vi "2283_controlDeElevador.vi"(0 "Cluster Niveles":T1) -> (2 "Output elevador":dbl)   [LabVIEW 2014]
uses:
  <vilib>/Rock Robotics/WPI/Solenoid/WPI_SolenoidValue.ctl
  Secuencia de Recoger Control.ctl
  DevRefs Global.vi
  Grip Overwrite Global.vi
  Cuernitos Global.vi
panel:
  in  "Margen de Error Secuencia de Recoger":dbl=50.0 format="%#_13g"
  in  "Nivel Cargar":dbl=60.0 format="%#_13g"
  in  "Nivel 1 Caja":dbl=225.0 format="%#_13g"
  in  "Nivel 2 Cajas":dbl=385.0 format="%#_13g"
  in  "Nivel 3 Cajas":dbl=607.0 format="%#_13g"
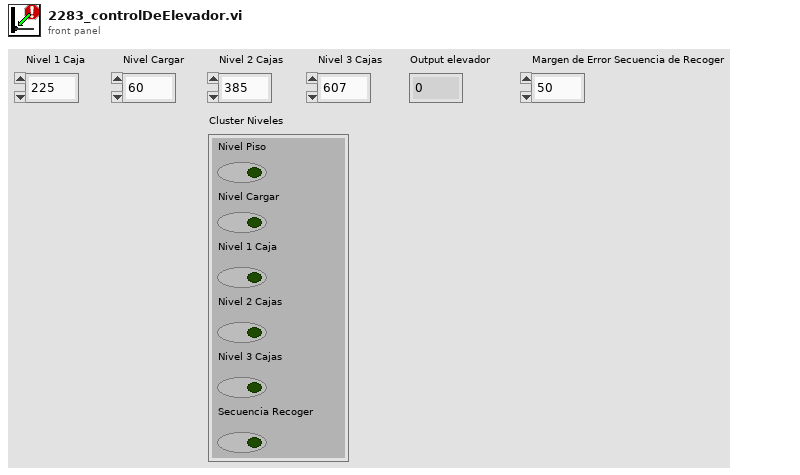
[diagram p1: front panel]
types:
  T1 = cluster{"Nivel Piso":bool, "Nivel Cargar":bool, "Nivel 1 Caja":bool, "Nivel 2 Cajas":bool, "Nivel 3 Cajas":bool, "Secuencia Recoger":bool}
  T2 = typedef "WPI_SolenoidDevRef.ctl" = cluster{"DevStatus":errorcluster, "Pneumatics Control Module":u8, "Forward Solenoid Channel":T3, "Reverse Solenoid Channel":T3}
  T3 = typedef "WPI_SolenoidChannel.ctl" = enum8{"Solenoid 0", "Solenoid 1", "Solenoid 2", "Solenoid 3", "Solenoid 4", "Solenoid 5", "Solenoid 6", "Solenoid 7", "Invalid"}
  T4 = typedef "WPI_MotorControlDeviceRef.ctl" = cluster{"DeviceStatus":errorcluster, "Type":T5, "PWM":cluster{"Controller":T6, "PWM Channel":T7, "DeadBand":T8}, "CAN":cluster{"Device Number":u8, "Control Mode":T9, "Semaphore":T10, "Max Vout":dbl, "TalonSRX Control Mode":T11}, "Invert":bool, "TransformRef":T12, "InvTransformRef":T12}
  T5 = typedef "WPI_MotorControlType.ctl" = enum16{"PWM", "CAN", "CANTalonSRX"}
  T6 = typedef "FPGA_TypedefDigitalModule.ctl" = enum16{"Controller 1"}
  T7 = typedef "FPGA_DIOPWMChannel.ctl" = enum8{"PWM 0", "PWM 1", "PWM 2", "PWM 3", "PWM 4", "PWM 5", "PWM 6", "PWM 7", "PWM 8", "PWM 9", "PWM MXP 0", "PWM MXP 1", "PWM MXP 2", "PWM MXP 3", "PWM MXP 4", "PWM MXP 5", "PWM MXP 6", "PWM MXP 7", "PWM MXP 8", "PWM MXP 9", "Invalid"}
  T8 = typedef "WPI_PWMDeadband.ctl" = cluster{"Name":string, "maxPositivePwm":i32, "minPositivePwm":i32, "centerPwm":i32, "maxNegativePwm":i32, "minNegativePwm":i32, "angularRange":u16}
  T9 = typedef "WPI_CANJaguar_ControlMode.ctl" = enum8{"Percent VBus", "Current", "Speed", "Position", "Voltage"}
  T10 = typedef "Semaphore RefNum" = refnum<k1>
  T11 = typedef "WPI_CANTalonSRX_APIControlMode.ctl" = enum8{"Percent VBus", "Speed", "Position", "Slave", "Unchanged / Invalid"}
  T12 = typedef "WPI_PWMTransform_ConPane.ctl" = refnum<vi>
  T13 = typedef "WPI_CompressorDevRef.ctl" = cluster{"DevStatus":errorcluster, "Pneumatics Control Module":u8}
  T14 = typedef "WPI_SwitchDevRef.ctl" = cluster{"DevStatus":errorcluster, "DIO Channel":T15, "Controller":T6, "CntIndex":T16, "Normally Closed":bool}
  T15 = typedef "FPGA_DIOChannel.ctl" = enum8{"DIO 0", "DIO 1", "DIO 2", "DIO 3", "DIO 4", "DIO 5", "DIO 6", "DIO 7", "DIO 8", "DIO 9", "DIO MXP 0", "DIO MXP 1", "DIO MXP 2", "DIO MXP 3", "DIO MXP 4", "DIO MXP 5", "DIO MXP 6", "DIO MXP 7", "DIO MXP 8", "DIO MXP 9", "DIO MXP 10", "DIO MXP 11", "DIO MXP 12", "DIO MXP 13", "DIO MXP 14", "DIO MXP 15", "Invalid"}
  T16 = typedef "FPGA_CounterCtrSystemIndex.ctl" = enum8{"Ctr 0", "Ctr 1", "Ctr 2", "Ctr 3", "Ctr 4", "Ctr 5", "Ctr 6", "Ctr 7", "Invalid"}
  T17 = typedef "WPI_GyroDevRef.ctl" = cluster{"DevStatus":errorcluster, "Analog Module":T18, "Analog Channel":T19, "Offset":dbl, "Gain (VoltsPerDegree/Second)":dbl}
  T18 = typedef "FPGA_TypedefAnalogModule.ctl" = enum16{"Controller 1"}
  T19 = typedef "FPGA_AIChannel.ctl" = enum8{"AI 0", "AI 1", "AI 2", "AI 3", "AI MXP 0", "AI MXP 1", "AI MXP 2", "AI MXP 3", "Invalid"}
  T20 = typedef "WPI_JoystickDevRef.ctl" = cluster{"Device":T21}
  T21 = typedef "WPI_JoystickDeviceEnum.ctl" = enum16{"USB 0", "USB 1", "USB 2", "USB 3", "USB 4", "USB 5"}
  T22 = typedef "WPI_AccelerometerDevRef.ctl" = cluster{"DevStatus":errorcluster, "Controller":T18, "Scaling":T23, "Analog Channels":T24, "I2C Bus":T25, "SPI Bus":T26, "Accel Range":T27, "ADXL345 Axes":T28, "Handle":i32, "Device Address":u8, "Accel Type":enum16{"Analog", "ADXL345 I2C", "ADXL345 SPI", "Internal"}}
  T23 = typedef "WPI_AccelerometerScaling.ctl" = cluster{"Gain (VoltsPerG)":dbl, "Center Voltage":dbl}
  T24 = typedef "WPI_AccelerometerAnalogChannels.ctl" = cluster{"X-Axis":T19, "Y-Axis":T19, "Z-Axis":T19}
  T25 = typedef "i2c_bus.ctl" = enum16{"I2C On-Board", "I2C MXP", "Invalid"}
  T26 = typedef "spi_bus.ctl" = enum16{"SPI On-Board, CS0", "SPI On-Board, CS1", "SPI On-Board, CS2", "SPI On-Board, CS3", "SPI MXP", "Invalid"}
  T27 = typedef "ADXL345 Range.ctl" = u8
  T28 = typedef "WPI_AccelerometerADXL345 Axes.ctl" = cluster{"X-Axis":bool, "Y-Axis":bool, "Z-Axis":bool}
  T29 = typedef "WPI_ServoDeviceRef.ctl" = cluster{"DeviceStatus":errorcluster, "Controller":T6, "PWM Channel":T7, "DeadBand":T8}
  T30 = typedef "WPI_EncoderDevRef.ctl" = cluster{"DevStatus":errorcluster, "EncoderIndex":T31, "CounterIndex":T16, "DistancePerCount":dbl, "Decoding Type":T32}
  T31 = typedef "FPGA_EncoderIdx.ctl" = enum8{"Enc 0", "Enc 1", "Enc 2", "Enc 3", "Enc 4", "Enc 5", "Enc 6", "Enc 7", "Invalid"}
  T32 = typedef "WPI_EncoderType.ctl" = enum16{"1x", "2x", "4x"}
  T33 = typedef "WPI_I2CDevRef.ctl" = cluster{"DevStatus":errorcluster, "Controller":T6, "Device Address":u8, "Handle":i32, "I2C Bus":T25}
  T34 = cluster{"Solenoide Cuernito Izquierdo":T2, "Solenoide Cuernito Derecho":T2, "Gripper":T2, "CAN Derecho Adelante":T4, "CAN Derecho Atras":T4, "CAN Izquierdo Atras":T4, "CAN Izquierdo Adelante":T4, "Compresora":T13, "Elevador Abajo":T14, "Elevador Abajo 2":T14, "Elevador Arriba":T14, "Gyro 1":T17, "Gyro 2":T17, "Joystick":T20, "Driver Station":T20, "Motor Cuernito Derecho":T4, "Motor Cuernito Izquierdo":T4, "Acelerometro":T22, "Servo":T29, "Encoder Elevador":T30, "Motor 1 Elevador":T4, "Motor 2 Elevador":T4, "Arduino I2C":T33, "LIDAR I2C":T33}
  T35 = typedef "WPI_SolenoidValue.ctl" = enum16{"Off", "On", "Forward", "Reverse"}
  T36 = typedef "Seleccion de Nivel Control.ctl" = enum16{"NA", "Nivel Piso", "Nivel Cargar", "Nivel 1 Caja", "Nivel 2 Cajas", "Nivel 3 Cajas", "Secuencia Recoger"}
  T37 = cluster{"Nivel Cargar":dbl, "Nivel 1 Caja":dbl, "Nivel 2 Cajas":dbl, "Nivel 3 Cajas":dbl}
  T38 = typedef "Secuencia de Recoger Control.ctl" = enum16{"Bajar a Suelo", "Abrir Cuernitos", "Subir a Cargar", "Stand-by"}
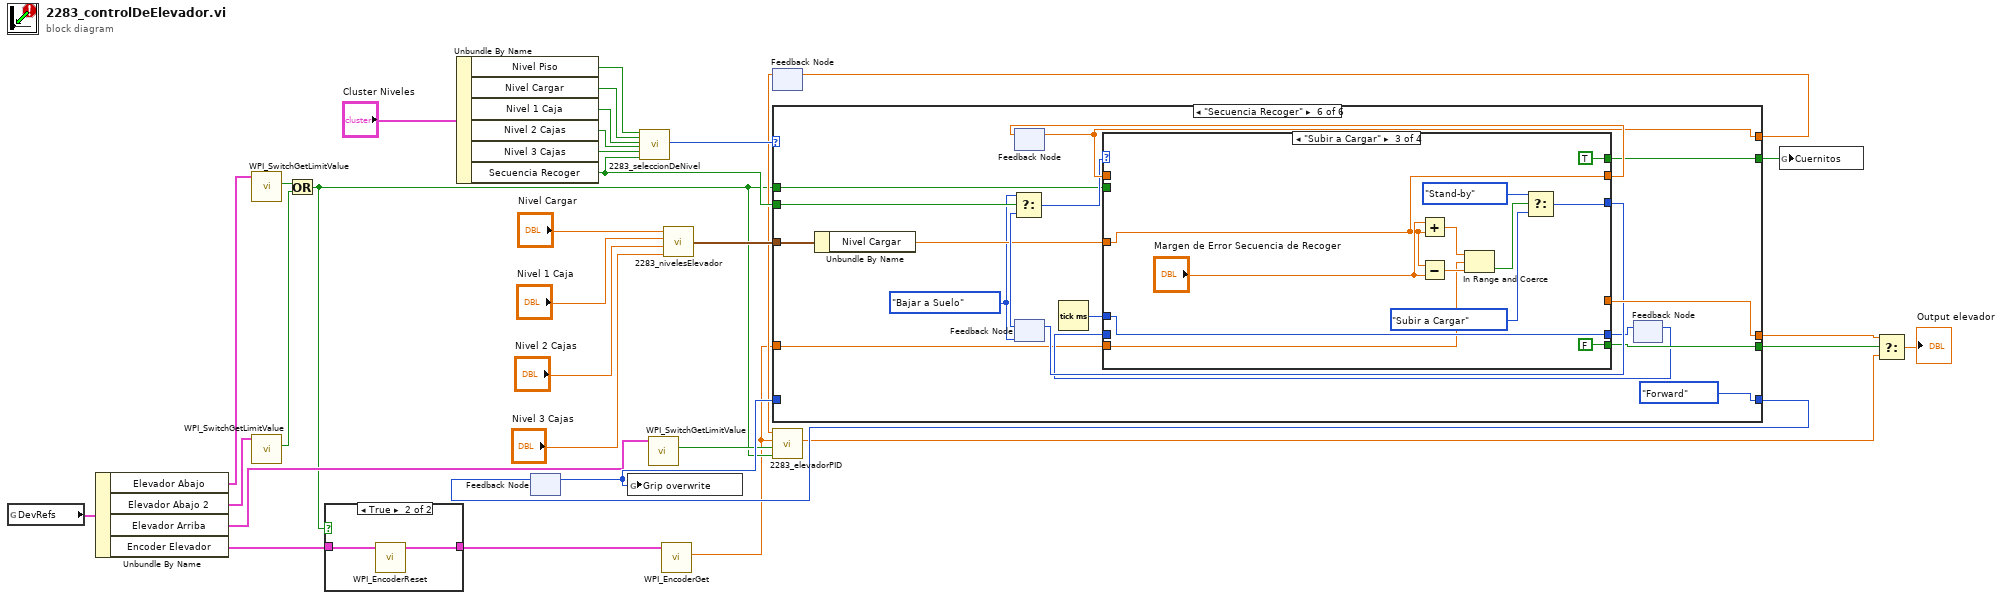
[diagram p0: block diagram]
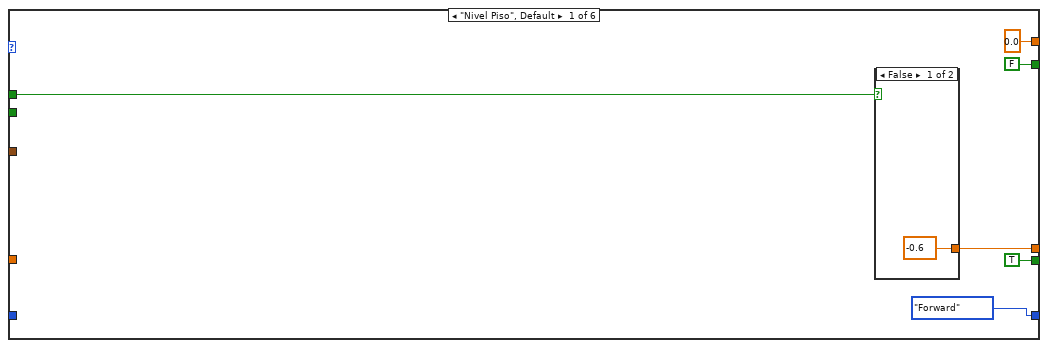
[diagram p2: hidden frame]
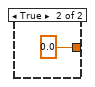
[diagram p3: hidden frame]
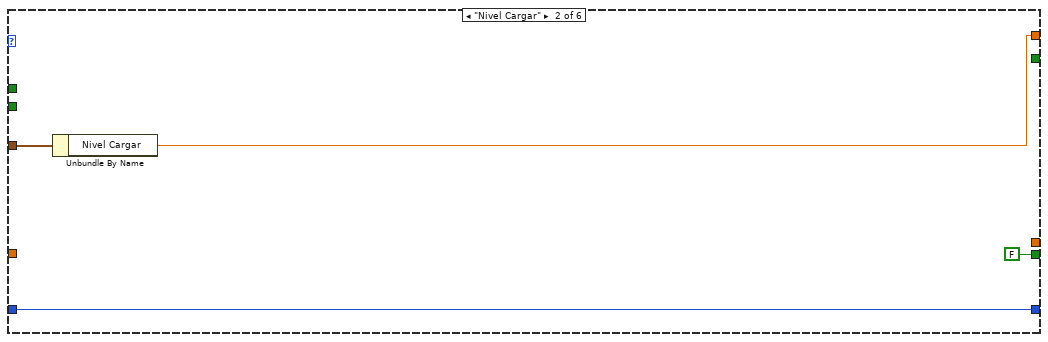
[diagram p4: hidden frame]
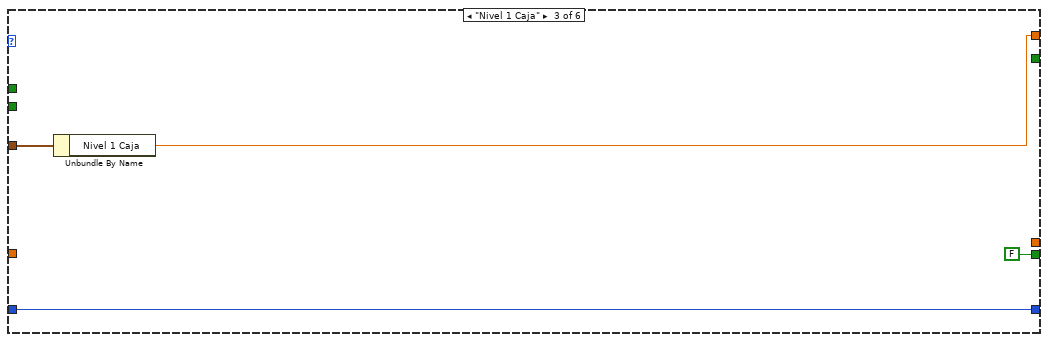
[diagram p5: hidden frame]
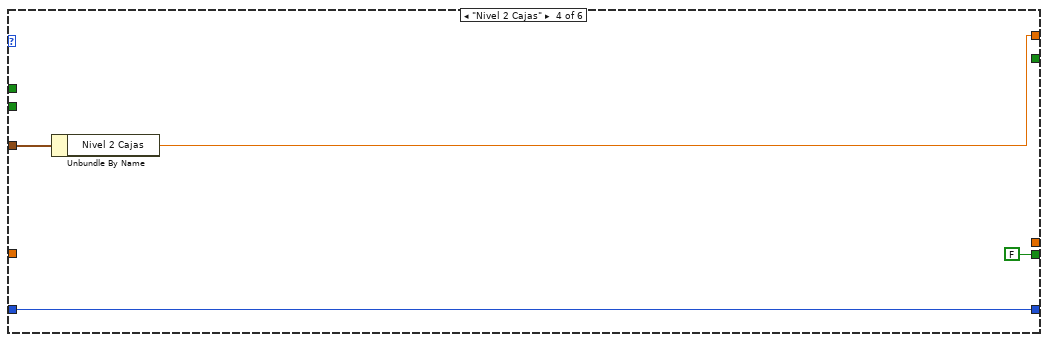
[diagram p6: hidden frame]
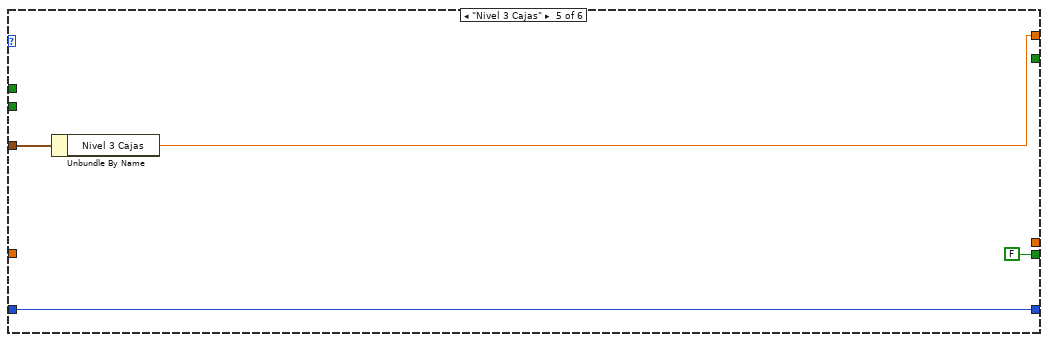
[diagram p7: hidden frame]
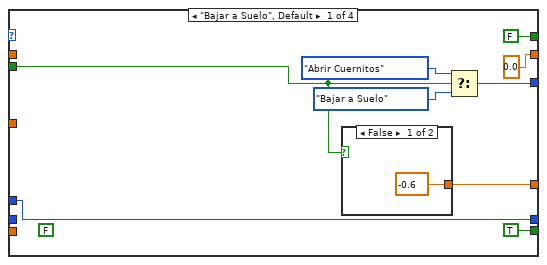
[diagram p8: hidden frame]
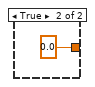
[diagram p9: hidden frame]
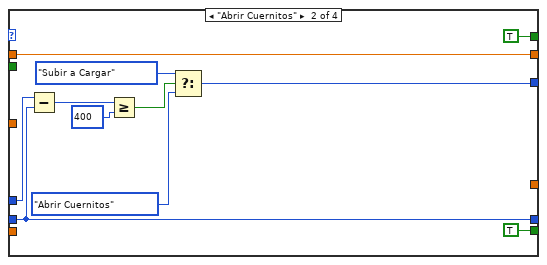
[diagram p10: hidden frame]
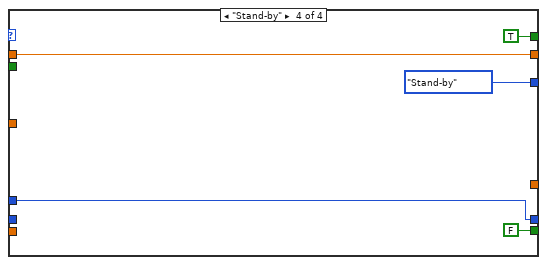
[diagram p11: hidden frame]
diagram:
  n1 = global read "DevRefs Global.vi" "DevRefs"() -> (w11:T34)
  n2 = Unbundle By Name(w11) -> ("Elevador Abajo"=w10:T14, "Elevador Abajo 2"=w9:T14, "Elevador Arriba"=w7:T14, "Encoder Elevador"=w6:T30)
  n3 = call <vilib>:"WPI_SwitchGetLimitValue.vi"("SwitchDevRef"=w10) -> ("Switch Pressed"=w22:bool)  [unwired: 8 in, 2 out]
  n4 = call <vilib>:"WPI_SwitchGetLimitValue.vi"("SwitchDevRef"=w9) -> ("Switch Pressed"=w8:bool)  [unwired: 8 in, 2 out]
  n5 = Or(x=w22, y=w8) -> (x .or. y?=w2:bool)
  n6 = case shown="True" w2 {
    tunnel: w6 -> [w34 w36]
    tunnel: [w34 w35] -> w33
    frame False {
    }
    frame True {
      n7 = call <vilib>:"WPI_EncoderReset.vi"("EncoderDevRef"=w36) -> ("EncoderDevRef"=w35:T30)  [unwired: 9 in, 1 out]
    }
  }
  n8 = Unbundle By Name("Cluster Niveles") -> ("Nivel Piso"=w17:bool, "Nivel Cargar"=w16:bool, "Nivel 1 Caja"=w15:bool, "Nivel 2 Cajas"=w14:bool, "Nivel 3 Cajas"=w13:bool, "Secuencia Recoger"=w12:bool)
  n9 = feedback #1() -> (w23:T35)  [unwired: 1 in]
  n10 = global write "Grip Overwrite Global.vi" "Grip overwrite"(w23) -> ()
  n11 = call "2283_seleccionDeNivel.vi"("Nivel Piso"=w17, "Nivel Cargar"=w16, "Nivel 1 Caja"=w15, "Nivel 2 Cajas"=w14, "Nivel 3 Cajas"=w13, "Secuencia Recoger"=w12) -> ("Nivel Deseado"=w18:T36)  [unwired: 13 in]
  n12 = call <vilib>:"WPI_SwitchGetLimitValue.vi"("SwitchDevRef"=w7) -> ("Switch Pressed"=w3:bool)  [unwired: 8 in, 2 out]
  n13 = call <vilib>:"WPI_EncoderGet.vi"("EncoderDevRef"=w33) -> ("Distance"=w1:dbl)  [unwired: 5 in, 5 out]
  n14 = call "2283_nivelesElevador.vi"("Nivel 3 cajas"="Nivel 3 Cajas", "Nivel 2 cajas"="Nivel 2 Cajas", "Nivel 1 caja"="Nivel 1 Caja", "Nivel cargar"="Nivel Cargar") -> ("output cluster"=w19:T37)
  n15 = feedback #2() -> (w4:dbl)  [unwired: 1 in]
  n16 = case shown="\"Secuencia Recoger\"" w18 {
    tunnel: [0.0 ("Nivel 1 caja") w47 w50 w54 w57 w75] -> w27
    tunnel: [w41 _ _ _ _ w78] -> w26
    tunnel: [FALSE _ _ _ _ w67] -> w21
    tunnel: [TRUE FALSE FALSE FALSE FALSE w72] -> w20
    tunnel: w12 -> [_ _ _ _ _ w68]
    tunnel: [WPI_SolenoidValue."Forward" ("Value") w48 w52 w56 w60 WPI_SolenoidValue."Forward" ("Value")] -> w24
    tunnel: w23 -> [_ w48 w52 w56 w60 _]
    tunnel: w19 -> [_ w46 w49 w55 w58 w65]
    tunnel: w2 -> [w37 _ _ _ _ w62]
    tunnel: w1 -> [_ _ _ _ _ w61]
    frame "Nivel Piso", Default {
      n17 = case shown="False" w37 {
        tunnel: [-0.6 ("upper limit") 0.0 ("upper limit")] -> w41
        frame False {
        }
        frame True {
        }
      }
    }
    frame "Nivel Cargar" {
      n18 = Unbundle By Name(w46) -> ("Nivel Cargar"=w47:dbl)
    }
    frame "Nivel 1 Caja" {
      n19 = Unbundle By Name(w49) -> ("Nivel 1 Caja"=w50:dbl)
    }
    frame "Nivel 2 Cajas" {
      n20 = Unbundle By Name(w55) -> ("Nivel 2 Cajas"=w54:dbl)
    }
    frame "Nivel 3 Cajas" {
      n21 = Unbundle By Name(w58) -> ("Nivel 3 Cajas"=w57:dbl)
    }
    frame "Secuencia Recoger" {
      w63 = Secuencia_de_Recoger_Control."Bajar a Suelo"
      n22 = Unbundle By Name(w65) -> ("Nivel Cargar"=w64:dbl)
      n23 = feedback #3() -> (w75:dbl)  [unwired: 1 in]
      n24 = feedback #4(w63) -> (w74:T38)
      n25 = Select(t=w63, s=w68, f=w74) -> (s? t:f=w73:T38)
      n26 = Tick Count (ms)() -> (millisecond timer value=w69:u32)
      n27 = feedback #5() -> (w70:u32)  [unwired: 1 in]
      n28 = case shown="\"Subir a Cargar\"" w73 {
        tunnel: w64 -> [_ _ w104 _]
        tunnel: [0.0 ("Nivel 1 caja") w100 w104 w113] -> w76
        tunnel: [w87 _ _ _] -> w78
        tunnel: [w86 w99 w108 Secuencia_de_Recoger_Control."Stand-by"] -> w77
        tunnel: w75 -> [_ w100 _ w113]
        tunnel: [FALSE ("Cuernitos") TRUE ("Cuernitos") TRUE ("Cuernitos") TRUE ("Cuernitos")] -> w67
        tunnel: [TRUE TRUE FALSE FALSE] -> w72
        tunnel: [w82 w93 w105 w116] -> w71
        tunnel: w70 -> [_ w93 _ _]
        tunnel: w69 -> [w82 w95 w105 w116]
        tunnel: w62 -> [w79 _ _ _]
        tunnel: w61 -> [_ _ w101 _]
        frame "Bajar a Suelo", Default {
          (unwired) FALSE
          n29 = case shown="False" w79 {
            tunnel: [-0.6 ("upper limit") 0.0 ("upper limit")] -> w87
            frame False {
            }
            frame True {
            }
          }
          n30 = Select(t=Secuencia_de_Recoger_Control."Abrir Cuernitos", s=w79, f=Secuencia_de_Recoger_Control."Bajar a Suelo") -> (s? t:f=w86:T38)
        }
        frame "Abrir Cuernitos" {
          n31 = Subtract(x=w95, y=w93) -> (x-y=w97:u32)
          n32 = Greater Or Equal?(x=w97, y=u32 400) -> (x >= y?=w94:bool)
          n33 = Select(t=Secuencia_de_Recoger_Control."Subir a Cargar", s=w94, f=Secuencia_de_Recoger_Control."Abrir Cuernitos") -> (s? t:f=w99:T38)
        }
        frame "Subir a Cargar" {
          n34 = Add(x="Margen de Error Secuencia de Recoger", y=w104) -> (x+y=w110:dbl)
          n35 = Subtract(x=w104, y="Margen de Error Secuencia de Recoger") -> (x-y=w112:dbl)
          n36 = In Range and Coerce(upper limit=w110, x=w101, lower limit=w112) -> (In Range?=w109:bool)  [unwired: 1 out]
          n37 = Select(t=Secuencia_de_Recoger_Control."Stand-by", s=w109, f=Secuencia_de_Recoger_Control."Subir a Cargar") -> (s? t:f=w108:T38)
        }
        frame "Stand-by" {
        }
      }
      n38 = feedback-in #3(w76) -> ()
      n39 = feedback-in #4(w77) -> ()
      n40 = feedback-in #5(w71) -> ()
    }
  }
  n41 = feedback-in #1(w24) -> ()
  n42 = feedback-in #2(w27) -> ()
  n43 = call "2283_elevadorPID.vi"("Tocando Switch abajo"=w2, "Tocando Switch Arriba"=w3, "process variable"=w1, "setpoint"=w4) -> ("Output Elevador"=w5:dbl)  [unwired: 7 in]
  n44 = global write "Cuernitos Global.vi" "Cuernitos"(w21) -> ()
  n45 = Select(t=w26, s=w20, f=w5) -> (s? t:f=→"Output elevador":dbl)
